vi "Normalize.vi"() -> ()   [LabVIEW 2018]
panel:
  out "A1":dbl
  in  "Min":dbl
  in  "Max":dbl
  out "A0":dbl
  in  "stop":bool
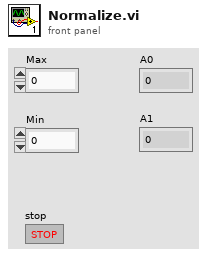
[diagram p1: front panel]
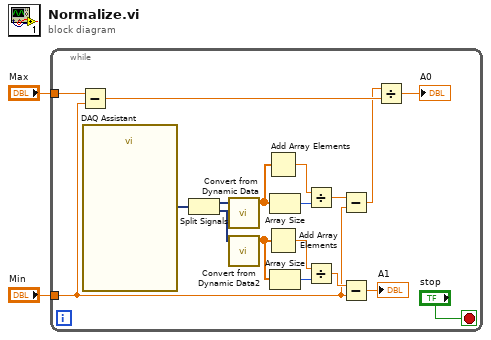
[diagram p0: block diagram]
diagram:
  n1 = while {
    tunnel: "Max" -> [w13]
    tunnel: "Min" -> [w4]
    stop <- "stop" stop-if-true
    n2 = Subtract(x=w13, y=w4) -> (x-y=w12:dbl)
    n3 = call "DAQ Assistant"() -> ("data"=w20:dynamicdata)  [unwired: 17 in, 2 out]
    n4 = Split Signals(w20) -> (w18:dynamicdata, w6:dynamicdata)  [unwired: 2 in]
    n5 = call "Convert from Dynamic Data"("Dynamic Data Type"=w18) -> ("Array"=w14:dbl[])  [unwired: 3 in]
    n6 = call "Convert from Dynamic Data2"("Dynamic Data Type"=w6) -> ("Array"=w7:dbl[])  [unwired: 3 in]
    n7 = Add Array Elements(numeric array=w14) -> (sum=w17:dbl)
    n8 = Add Array Elements(numeric array=w7) -> (sum=w9:dbl)
    n9 = Array Size(array=w14) -> (size(s)=w16:i32)
    n10 = Array Size(array=w7) -> (size(s)=w8:i32)
    n11 = Divide(x=w17, y=w16) -> (x/y=w11:dbl)
    n12 = Divide(x=w9, y=w8) -> (x/y=w5:dbl)
    n13 = Subtract(x=w11, y=w4) -> (x-y=w10:dbl)
    n14 = Subtract(x=w5, y=w4) -> (x-y=→"A1":dbl)
    n15 = Divide(x=w10, y=w12) -> (x/y=→"A0":dbl)
  }
